vi "celiang2.vi"(7 "error in":errorcluster) -> (27 "error out":errorcluster)   [LabVIEW 2014]
uses:
  <vilib>/vision/Image Controls.llb/Vision Info Type2.ctl
  <vilib>/vision/NI_Vision_Development_Module.lvlib
panel:
  out "Image Out":T1(plugin-control)
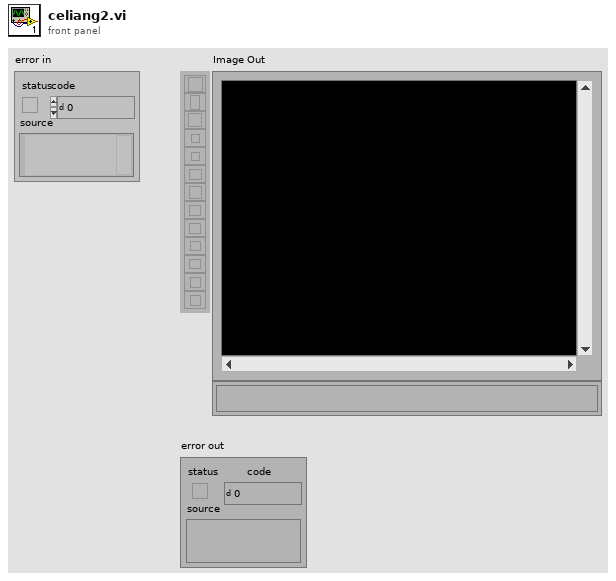
[diagram p1: front panel]
types:
  T1 = typedef "IMAQ Image.ctl" = refnum<image>
  T2 = cluster{"Contrast":i32, "Filter width":i32, "Steepness":i32, "Subsampling Ratio":u32, "Show Search Area":bool, "Show Search Lines":bool, "Show Edges Found":bool, "Show Result":bool}
  T3 = cluster{"Global Rectangle":i32[], "Contours":cluster{"ID":enum32{"External", "Internal"}, "Type":u32, "Coordinates":i32[]}[]}
  T4 = cluster{"Origin":cluster{"X":sgl, "Y":sgl}, "Angle (deg)":sgl, "Axis Reference":u32}
  T5 = enum16{"Reset", "Update Coordinate System", "Get Coordinate System"}
  T6 = enum16{"Horizontal Motion", "Vertical Motion", "Horizontal and Vertical Motion", "Horizontal, Vertical and Angular Motion"}
  T7 = enum16{"Get First Edge", "Get First + Last Edge", "Get All Edges"}
  T8 = cluster{"Level Type":enum32{"Absolute Value", "Relative value"}, "Threshold Level":i32, "Hysteresis":i32}
  T9 = cluster{"Origin Pixel":cluster{"X":sgl, "Y":sgl}, "X Axis Pixel":cluster{"X":sgl, "Y":sgl}, "Axis Reference":u32}
  T10 = typedef "Vision Info Type2.ctl" = u32
  T11 = typedef "Simple Grid Descriptor" = cluster{"X Step":sgl, "Y Step":sgl, "Unit":T12}
  T12 = typedef "Image Unit" = enum32{"Undefined", "Angström", "Micrometer", "Millimeter", "Centimeter", "Meter", "Kilometer", "Microinch", "Inch", "Feet", "Nautical miles", "Standard miles", "Steps"}
  T13 = typedef "Image Type" = u32
  T14 = typedef "IMAQ Coordinate System" = cluster{"Reference System":cluster{"Origin":cluster{"X":sgl, "Y":sgl}, "Angle (deg)":sgl, "Axis Reference":u32}, "Measurement System":cluster{"Origin":cluster{"X":sgl, "Y":sgl}, "Angle (deg)":sgl, "Axis Reference":u32}}
  T15 = typedef "ROI Descriptor" = cluster{"Global Rectangle":i32[], "Contours":cluster{"ID":enum32{"External", "Internal"}, "Type":u32, "Coordinates":i32[]}[]}
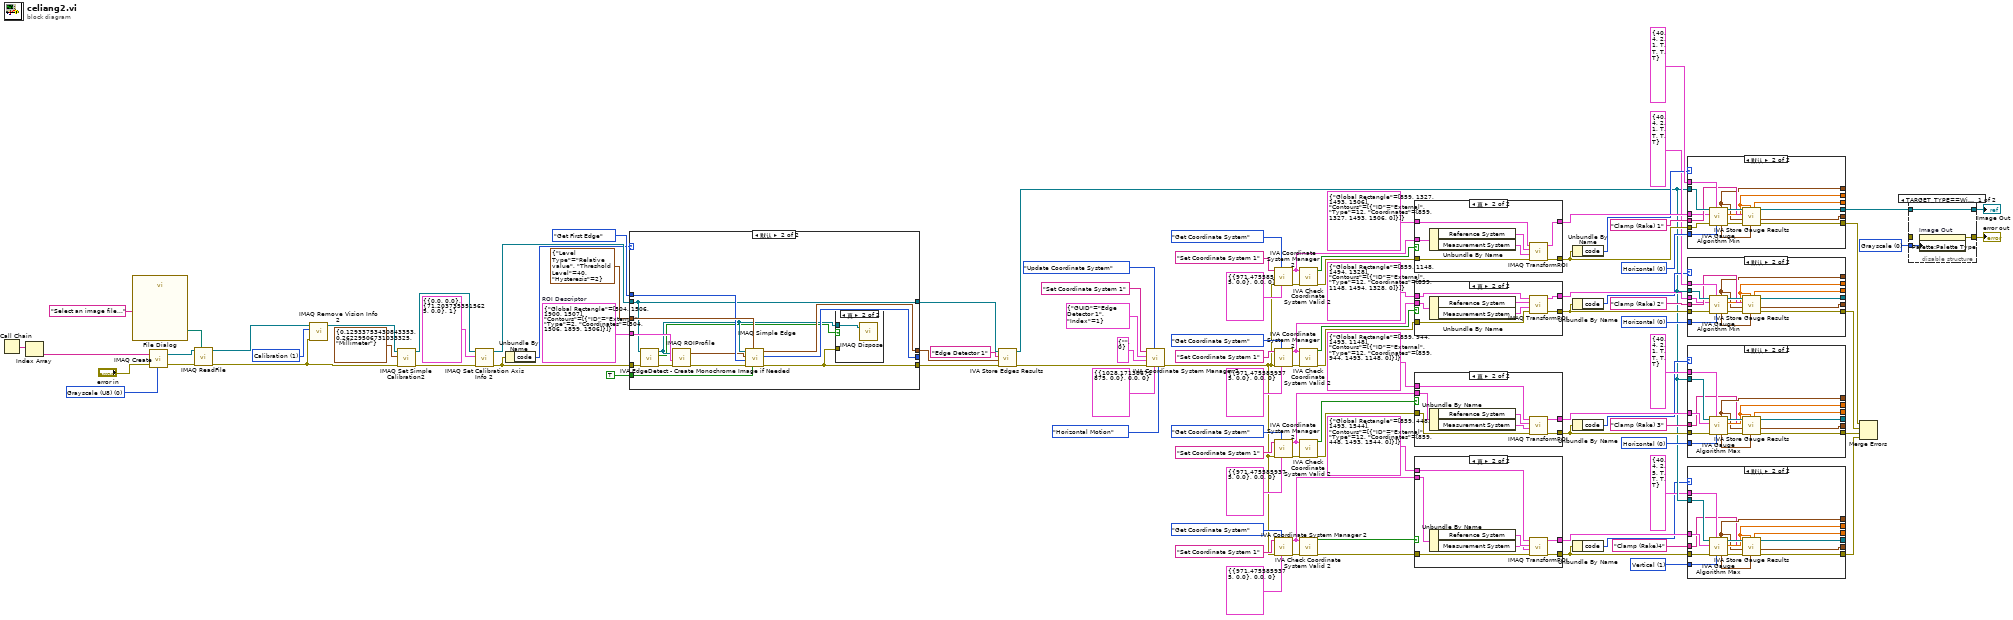
[diagram p0: block diagram]
diagram:
  w1 = u32 0 items=["Grayscale", "Binary", "Gradient", "Rainbow", "Temperature", "User Defined"] ("Palette")
  w13 = u32 1 items=["Horizontal", "Vertical"] ("Scanning axis")
  w29 = u32 0 items=["Horizontal", "Vertical"] ("Scanning axis")
  w41 = u32 0 items=["Horizontal", "Vertical"] ("Scanning axis")
  w55 = u32 0 items=["Horizontal", "Vertical"] ("Scanning axis")
  w78 = T3 {"Global Rectangle"=[504, 1506, 1900, 1507], "Contours"=[{"ID"=enum."External", "Type"=2, "Coordinates"=[504, 1506, 1899, 1506]}]}  # ROI Descriptor
  w91 = T10 1 items=["Any", "Calibration", "Overlay", "Grayscale Template", "Color Template", "Geometric Template", "Custom Data", "Golden Template", "Geometric Template 2", "Contour Data", "Camera Model"] ("Vision Info")
  w93 = T13 0 items=["Grayscale (U8)", "Grayscale (I16)", "Grayscale (SGL)", "Complex (CSG)", "RGB (U32)", "HSL (U32)", "RGB (U64)", "Grayscale (U16)"] ("Image Type")
  n1 = Call Chain() -> (call chain=w97:string[])
  n2 = Index Array(array=w97) -> (element=w96:string)  [unwired: 1 in]
  n3 = call "File Dialog"("prompt"="Select an image file...") -> ("selected path"=w94:path)  [unwired: 6 in, 8 out]
  n4 = call "IMAQ Create"("Image Name"=w96, "Image Type"=w93, "error in (no error)"="error in") -> ("New Image"=w100:T1, "error out"=w99:errorcluster)  [unwired: 1 in, 1 out]
  n5 = call "IMAQ ReadFile"("File Path"=w94, "error in (no error)"=w99, "Image"=w100) -> ("error out"=w88:errorcluster, "Image Out"=w90:T1)  [unwired: 2 in, 5 out]
  n6 = call "IMAQ Remove Vision Info 2"("error in (no error)"=w88, "Vision Info"=w91, "Image"=w90) -> ("Image Out"=w89:T1)  [unwired: 8 out]
  n7 = call "IMAQ Set Simple Calibration2"("error in (no error)"=w88, "Pixel Distances"=T11 {"X Step"=0.12933753, "Y Step"=0.26229507, "Unit"=enum."Millimeter"} ("Grid Descriptor"), "Image"=w89) -> ("error out"=w86:errorcluster, "Calibration Template Image"=w87:T1)  [unwired: 2 in, 5 out]
  n8 = call-poly "IMAQ Set Calibration Axis Info 2"("error in (no error)"=w86, "Calibration Axis Info"=T9 {"Origin Pixel"={"X"=0.0, "Y"=0.0}, "X Axis Pixel"={"X"=71.203735, "Y"=0.0}, "Axis Reference"=1}, "Calibration Template Image In"=w87) -> ("error out"=w77:errorcluster, "Calibration Template Image Out"=w82:T1)  [unwired: 7 out]
  n9 = Unbundle By Name(w77) -> ("code"=w76:i32)
  n10 = case "条件结构" shown="默认" w76 {
    tunnel: T8 {"Level Type"=enum."Relative value", "Threshold Level"=40, "Hysteresis"=2} ("Threshold Parameters") -> [_ w115]
    tunnel: T7."Get First Edge" ("Process") -> [_ w114]
    tunnel: [_ w113] -> _
    tunnel: w77 -> [_ w106]
    tunnel: w82 -> [w101 w107]
    tunnel: [_ w110] -> w80
    tunnel: [_ w102] -> w79
    tunnel: w78 -> [_ w109]
    tunnel: TRUE ("Sub-Pixel Accuracy") -> [_ w108]
    tunnel: [w101 w107] -> w74
    frame -1074396199, -1074396198 {
      # "Discard Coordinate System Error"
    }
    frame Default {
      n11 = call <vilib>:"IVA EdgeDetect - Create Monochrome Image if Needed.vi"("error in (no error)"=w106, "Image In"=w107) -> ("error out"=w105:errorcluster, "Mono Image Created"=w103:bool, "Mono Image Out"=w104:T1)  [unwired: 7 out]
      n12 = call "IMAQ ROIProfile"("error in (no error)"=w105, "ROI Descriptor"=w109, "Image"=w104) -> ("error out"=w111:errorcluster, "Pixel Coordinates"=w112:cluster{"X":u32, "Y":u32}[])  [unwired: 4 out]
      n13 = call "IMAQ Simple Edge"("Sub-Pixel Accuracy"=w108, "Threshold Parameters"=w115, "error in (no error)"=w111, "Process"=w114, "Pixel Coordinates"=w112, "Image Src"=w104) -> ("error out"=w102:errorcluster, "Number of Edges"=w113:i32, "Edges Coordinates"=w110:cluster{"X":sgl, "Y":sgl}[])  [unwired: 3 out]
      n14 = case "条件结构" shown="真" w103 {
        tunnel: w104 -> [_ w116]
        tunnel: w102 -> [_ _]
        frame False {
        }
        frame True {
          n15 = call "IMAQ Dispose"("Image"=w116) -> ()  [unwired: 2 in, 4 out]
        }
      }
    }
  }
  n16 = call <vilib>:"IVA Store Edges Results.vi"("error in (no error)"=w79, "Edge Coordinates"=w80, "Step Name"="Edge Detector 1", "Image in"=w74) -> ("error out"=w67:errorcluster, "Image dup"=w15:T1)  [unwired: 6 out]
  n17 = call <vilib>:"IVA Coordinate System Manager 2.vi"("Mode"=T6."Horizontal Motion", "Reference System"=T4 {"Origin"={"X"=1028.1714, "Y"=0.0}, "Angle (deg)"=0.0, "Axis Reference"=0}, "Function"=T5."Update Coordinate System", "error in (no error)"=w67, "Angle ID"=cluster{"GUID":string, "Index":i32} {"GUID"="", "Index"=0}, "Origin ID"=cluster{"GUID":string, "Index":i32} {"GUID"="Edge Detector 1", "Index"=1}, "Coordinate System Name"="Set Coordinate System 1") -> ("error out"=w22:errorcluster)  [unwired: 4 out]
  n18 = call <vilib>:"IVA Coordinate System Manager 2.vi"("Reference System"=T4 {"Origin"={"X"=971.4756, "Y"=0.0}, "Angle (deg)"=0.0, "Axis Reference"=0}, "Function"=T5."Get Coordinate System", "error in (no error)"=w22, "Coordinate System Name"="Set Coordinate System 1") -> ("error out"=w60:errorcluster, "Coordinate System Out"=w62:T14)  [unwired: 3 in, 3 out]
  n19 = call <vilib>:"IVA Coordinate System Manager 2.vi"("Reference System"=T4 {"Origin"={"X"=971.4756, "Y"=0.0}, "Angle (deg)"=0.0, "Axis Reference"=0}, "Function"=T5."Get Coordinate System", "error in (no error)"=w22, "Coordinate System Name"="Set Coordinate System 1") -> ("error out"=w46:errorcluster, "Coordinate System Out"=w48:T14)  [unwired: 3 in, 3 out]
  n20 = call <vilib>:"IVA Coordinate System Manager 2.vi"("Reference System"=T4 {"Origin"={"X"=971.4756, "Y"=0.0}, "Angle (deg)"=0.0, "Axis Reference"=0}, "Function"=T5."Get Coordinate System", "error in (no error)"=w22, "Coordinate System Name"="Set Coordinate System 1") -> ("error out"=w32:errorcluster, "Coordinate System Out"=w34:T14)  [unwired: 3 in, 3 out]
  n21 = call <vilib>:"IVA Coordinate System Manager 2.vi"("Reference System"=T4 {"Origin"={"X"=971.4756, "Y"=0.0}, "Angle (deg)"=0.0, "Axis Reference"=0}, "Function"=T5."Get Coordinate System", "error in (no error)"=w22, "Coordinate System Name"="Set Coordinate System 1") -> ("error out"=w17:errorcluster, "Coordinate System Out"=w19:T14)  [unwired: 3 in, 3 out]
  n22 = call <vilib>:"IVA Check Coordinate System Valid 2.vi"("error in (no error)"=w60, "Coordinate System"=w62) -> ("error out"=w59:errorcluster, "Valid?"=w61:bool)  [unwired: 8 out]
  n23 = call <vilib>:"IVA Check Coordinate System Valid 2.vi"("error in (no error)"=w46, "Coordinate System"=w48) -> ("error out"=w45:errorcluster, "Valid?"=w47:bool)  [unwired: 8 out]
  n24 = call <vilib>:"IVA Check Coordinate System Valid 2.vi"("error in (no error)"=w32, "Coordinate System"=w34) -> ("error out"=w31:errorcluster, "Valid?"=w33:bool)  [unwired: 8 out]
  n25 = call <vilib>:"IVA Check Coordinate System Valid 2.vi"("error in (no error)"=w17, "Coordinate System"=w19) -> ("error out"=w16:errorcluster, "Valid?"=w18:bool)  [unwired: 8 out]
  n26 = case "条件结构" shown="真" w61 {
    tunnel: T3 {"Global Rectangle"=[859, 1327, 1493, 1506], "Contours"=[{"ID"=enum."External", "Type"=12, "Coordinates"=[859, 1327, 1493, 1506, 0]}]} ("ROI Descriptor") -> [w118 w125]
    tunnel: [w118 w122] -> w56
    tunnel: [w117 w121] -> w54
    tunnel: w62 -> [_ w120]
    tunnel: w59 -> [w117 w119]
    frame False {
    }
    frame True {
      n27 = Unbundle By Name(w120) -> ("Reference System"=w124:T4, "Measurement System"=w123:T4)
      n28 = call "IMAQ TransformROI"("error in (no error)"=w119, "New Reference"=w123, "Base Reference"=w124, "ROI Descriptor"=w125) -> ("error out"=w121:errorcluster, "ROI Descriptor out"=w122:T15)  [unwired: 6 out]
    }
  }
  n29 = case "条件结构" shown="真" w47 {
    tunnel: T3 {"Global Rectangle"=[859, 1148, 1494, 1328], "Contours"=[{"ID"=enum."External", "Type"=12, "Coordinates"=[859, 1148, 1494, 1328, 0]}]} ("ROI Descriptor") -> [w127 w134]
    tunnel: [w127 w131] -> w42
    tunnel: [w126 w130] -> w40
    tunnel: w48 -> [_ w129]
    tunnel: w45 -> [w126 w128]
    frame False {
    }
    frame True {
      n30 = Unbundle By Name(w129) -> ("Reference System"=w133:T4, "Measurement System"=w132:T4)
      n31 = call "IMAQ TransformROI"("error in (no error)"=w128, "New Reference"=w132, "Base Reference"=w133, "ROI Descriptor"=w134) -> ("error out"=w130:errorcluster, "ROI Descriptor out"=w131:T15)  [unwired: 6 out]
    }
  }
  n32 = case "条件结构" shown="真" w33 {
    tunnel: T3 {"Global Rectangle"=[859, 944, 1493, 1148], "Contours"=[{"ID"=enum."External", "Type"=12, "Coordinates"=[859, 944, 1493, 1148, 0]}]} ("ROI Descriptor") -> [w136 w143]
    tunnel: [w136 w140] -> w28
    tunnel: [w135 w139] -> w27
    tunnel: w34 -> [_ w138]
    tunnel: w31 -> [w135 w137]
    frame False {
    }
    frame True {
      n33 = Unbundle By Name(w138) -> ("Reference System"=w142:T4, "Measurement System"=w141:T4)
      n34 = call "IMAQ TransformROI"("error in (no error)"=w137, "New Reference"=w141, "Base Reference"=w142, "ROI Descriptor"=w143) -> ("error out"=w139:errorcluster, "ROI Descriptor out"=w140:T15)  [unwired: 6 out]
    }
  }
  n35 = case "条件结构" shown="真" w18 {
    tunnel: T3 {"Global Rectangle"=[859, 448, 1493, 1544], "Contours"=[{"ID"=enum."External", "Type"=12, "Coordinates"=[859, 448, 1493, 1544, 0]}]} ("ROI Descriptor") -> [w145 w152]
    tunnel: [w145 w149] -> w12
    tunnel: [w144 w148] -> w11
    tunnel: w19 -> [_ w147]
    tunnel: w16 -> [w144 w146]
    frame False {
    }
    frame True {
      n36 = Unbundle By Name(w147) -> ("Reference System"=w151:T4, "Measurement System"=w150:T4)
      n37 = call "IMAQ TransformROI"("error in (no error)"=w146, "New Reference"=w150, "Base Reference"=w151, "ROI Descriptor"=w152) -> ("error out"=w148:errorcluster, "ROI Descriptor out"=w149:T15)  [unwired: 6 out]
    }
  }
  n38 = Unbundle By Name(w54) -> ("code"=w53:i32)
  n39 = Unbundle By Name(w40) -> ("code"=w39:i32)
  n40 = Unbundle By Name(w27) -> ("code"=w26:i32)
  n41 = Unbundle By Name(w11) -> ("code"=w10:i32)
  n42 = case "条件结构" shown="默认" w53 {
    tunnel: T2 {"Contrast"=40, "Filter width"=4, "Steepness"=2, "Subsampling Ratio"=1, "Show Search Area"=TRUE, "Show Search Lines"=TRUE, "Show Edges Found"=TRUE, "Show Result"=TRUE} ("Settings") -> [_ w168]
    tunnel: w15 -> [w153 w167]
    tunnel: w54 -> [_ w166]
    tunnel: [w153 w164] -> w3
    tunnel: [_ w162] -> w8
    tunnel: "Clamp (Rake) 1" ("Step Name") -> [_ w161]
    tunnel: [_ w160] -> _
    tunnel: [_ w158] -> _
    tunnel: [_ w157] -> _
    tunnel: w56 -> [_ w156]
    tunnel: w55 -> [_ w155]
    tunnel: [_ w154] -> _
    frame -1074396199, -1074396198 {
      # "Discard Coordinate System Error"
    }
    frame Default {
      n43 = call <vilib>:"IVA Gauge Algorithm Min.vi"("Scanning axis"=w155, "Settings"=w168, "error in (no error)"=w166, "ROI Descriptor"=w156, "Image"=w167) -> ("error out"=w163:errorcluster, "Distance"=w160:sgl, "Image Out"=w165:T1, "Distance Points"=w159:cluster{"X":sgl, "Y":sgl}[], "Edge Coordinates"=w158:cluster{"X":sgl, "Y":sgl}[])  [unwired: 1 in, 1 out]
      n44 = call <vilib>:"IVA Store Gauge Results.vi"("Distance Points"=w159, "Distance"=w160, "error in (no error)"=w163, "Points of Contact"=w158, "Step Name"=w161, "Image in"=w165) -> ("error out"=w162:errorcluster, "Points of Contact (calibrated)"=w154:cluster{"X":sgl, "Y":sgl}[], "Image dup"=w164:T1, "Distance (calibrated)"=w157:sgl)  [unwired: 2 out]
    }
  }
  n45 = case "条件结构" shown="默认" w39 {
    tunnel: T2 {"Contrast"=40, "Filter width"=4, "Steepness"=2, "Subsampling Ratio"=1, "Show Search Area"=TRUE, "Show Search Lines"=TRUE, "Show Edges Found"=TRUE, "Show Result"=TRUE} ("Settings") -> [_ w184]
    tunnel: w15 -> [w169 w183]
    tunnel: w40 -> [_ w182]
    tunnel: [w169 w180] -> _
    tunnel: [_ w178] -> w7
    tunnel: "Clamp (Rake) 2" ("Step Name") -> [_ w177]
    tunnel: [_ w176] -> _
    tunnel: [_ w174] -> _
    tunnel: [_ w173] -> _
    tunnel: w42 -> [_ w172]
    tunnel: w41 -> [_ w171]
    tunnel: [_ w170] -> _
    frame -1074396199, -1074396198 {
      # "Discard Coordinate System Error"
    }
    frame Default {
      n46 = call <vilib>:"IVA Gauge Algorithm Min.vi"("Scanning axis"=w171, "Settings"=w184, "error in (no error)"=w182, "ROI Descriptor"=w172, "Image"=w183) -> ("error out"=w179:errorcluster, "Distance"=w176:sgl, "Image Out"=w181:T1, "Distance Points"=w175:cluster{"X":sgl, "Y":sgl}[], "Edge Coordinates"=w174:cluster{"X":sgl, "Y":sgl}[])  [unwired: 1 in, 1 out]
      n47 = call <vilib>:"IVA Store Gauge Results.vi"("Distance Points"=w175, "Distance"=w176, "error in (no error)"=w179, "Points of Contact"=w174, "Step Name"=w177, "Image in"=w181) -> ("error out"=w178:errorcluster, "Points of Contact (calibrated)"=w170:cluster{"X":sgl, "Y":sgl}[], "Image dup"=w180:T1, "Distance (calibrated)"=w173:sgl)  [unwired: 2 out]
    }
  }
  n48 = case "条件结构" shown="默认" w26 {
    tunnel: w15 -> [w185 w200]
    tunnel: w27 -> [_ w199]
    tunnel: T2 {"Contrast"=40, "Filter width"=4, "Steepness"=2, "Subsampling Ratio"=1, "Show Search Area"=TRUE, "Show Search Lines"=TRUE, "Show Edges Found"=TRUE, "Show Result"=TRUE} ("Settings") -> [_ w198]
    tunnel: w29 -> [_ w197]
    tunnel: w28 -> [_ w196]
    tunnel: [w185 w194] -> _
    tunnel: [_ w192] -> w6
    tunnel: [_ w191] -> _
    tunnel: [_ w190] -> _
    tunnel: [_ w189] -> _
    tunnel: [_ w188] -> _
    tunnel: "Clamp (Rake) 3" ("Step Name") -> [_ w187]
    frame -1074396199, -1074396198 {
      # "Discard Coordinate System Error"
    }
    frame Default {
      n49 = call <vilib>:"IVA Gauge Algorithm Max.vi"("Scanning axis"=w197, "Settings"=w198, "error in (no error)"=w199, "ROI Descriptor"=w196, "Image"=w200) -> ("error out"=w193:errorcluster, "Distance"=w191:sgl, "Image Out"=w195:T1, "Distance Points"=w186:cluster{"X":sgl, "Y":sgl}[], "Points of Contact"=w190:cluster{"X":sgl, "Y":sgl}[])  [unwired: 1 in, 1 out]
      n50 = call <vilib>:"IVA Store Gauge Results.vi"("Distance Points"=w186, "Distance"=w191, "error in (no error)"=w193, "Points of Contact"=w190, "Step Name"=w187, "Image in"=w195) -> ("error out"=w192:errorcluster, "Points of Contact (calibrated)"=w188:cluster{"X":sgl, "Y":sgl}[], "Image dup"=w194:T1, "Distance (calibrated)"=w189:sgl)  [unwired: 2 out]
    }
  }
  n51 = case "条件结构" shown="默认" w10 {
    tunnel: w15 -> [w201 w216]
    tunnel: w11 -> [_ w215]
    tunnel: T2 {"Contrast"=40, "Filter width"=4, "Steepness"=2, "Subsampling Ratio"=5, "Show Search Area"=TRUE, "Show Search Lines"=TRUE, "Show Edges Found"=TRUE, "Show Result"=TRUE} ("Settings") -> [_ w214]
    tunnel: w13 -> [_ w213]
    tunnel: w12 -> [_ w212]
    tunnel: [w201 w210] -> _
    tunnel: [_ w208] -> w5
    tunnel: [_ w207] -> _
    tunnel: [_ w206] -> _
    tunnel: [_ w205] -> _
    tunnel: [_ w204] -> _
    tunnel: "Clamp (Rake)4" ("Step Name") -> [_ w203]
    frame -1074396199, -1074396198 {
      # "Discard Coordinate System Error"
    }
    frame Default {
      n52 = call <vilib>:"IVA Gauge Algorithm Max.vi"("Scanning axis"=w213, "Settings"=w214, "error in (no error)"=w215, "ROI Descriptor"=w212, "Image"=w216) -> ("error out"=w209:errorcluster, "Distance"=w207:sgl, "Image Out"=w211:T1, "Distance Points"=w202:cluster{"X":sgl, "Y":sgl}[], "Points of Contact"=w206:cluster{"X":sgl, "Y":sgl}[])  [unwired: 1 in, 1 out]
      n53 = call <vilib>:"IVA Store Gauge Results.vi"("Distance Points"=w202, "Distance"=w207, "error in (no error)"=w209, "Points of Contact"=w206, "Step Name"=w203, "Image in"=w211) -> ("error out"=w208:errorcluster, "Points of Contact (calibrated)"=w204:cluster{"X":sgl, "Y":sgl}[], "Image dup"=w210:T1, "Distance (calibrated)"=w205:sgl)  [unwired: 2 out]
    }
  }
  n54 = Merge Errors(w8, w7, w6, w5) -> ()  [unwired: 1 out]
  n55 = disable-structure "条件禁用结构" shown="TARGET_TYPE==Windows" {
    disable-tunnel: _ -> [_ w220]
    disable-tunnel: [w219 w220] -> w4
    disable-tunnel: w3 -> [w218 w221]
    disable-tunnel: [w218 w221] -> w2
    disable-tunnel: w1 -> [w217 _]
    frame condition #0 (active) {
      n56 = property on="Image Out" class="ImageControl"("Palette:Palette Type"=w217) -> (error out=w219:errorcluster)  [unwired: 2 in, 1 out]
    }
    frame condition #1 {
    }
  }
  "error out" <- w4
  "Image Out" <- w2
